vi "CFTS-Build.vi"() -> ()   [LabVIEW 2020]
uses:
  CFTS SubVIs/CFTS-Globals.vi
panel:
  out "Version":string="0.1-alpha.0"
  out "Progress Bar":u8(slide) caption="Error" scale=0.0..4.0
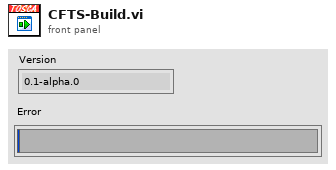
[diagram p1: front panel]
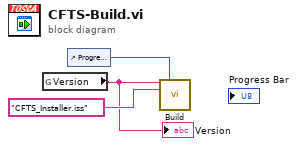
[diagram p0: block diagram]
diagram:
  n1 = global read "CFTS-Globals.vi" "Version"() -> (w1:string)
  "Version" <- w1
  n2 = control-ref of="Progress Bar"() -> (w3:refnum<vi>)
  n3 = call "Build.vi"("version"=w1, "Progress Bar"=w3, "iss path"="CFTS_Installer.iss") -> ()  [unwired: 13 in]
